vi "List Contents of Bucket.vi"() -> ()   [LabVIEW 2015]
doc: "This example shows you how to list the contents of your Amazon S3 bucket.\n\nThe list will contain information about all the objects you have in the bucket."
uses:
  <vilib>/AWS Toolkit/Core/HTTP Request/AWS Credentials.ctl
  <vilib>/AWS Toolkit/Core/HTTP Request/HTTP Request.lvclass
  <vilib>/AWS Toolkit/S3/Bucket/Bucket.lvclass
panel:
  in  "Bucket Name":string
  in  "Secret Key":string
  in  "Access Key":string
  out "Bucket Contents":i32(listbox)
  # "Overview: Demonstrates how to display the contents of an Amazon S3 bucket.\nRequirements: NI Cloud Toolkit for AWS and a registered Amazon AWS account\nInstructions:\n1. Specify the Access Key and Secret Key for your AWS account. You can create an account at http://aws.amazon.com.\n2. Specify a Bucket Name for the bucket you want to inspect.\n3. Run the VI. All of the contents of the specified bucket will be displayed in the Bucket Contents indicator."
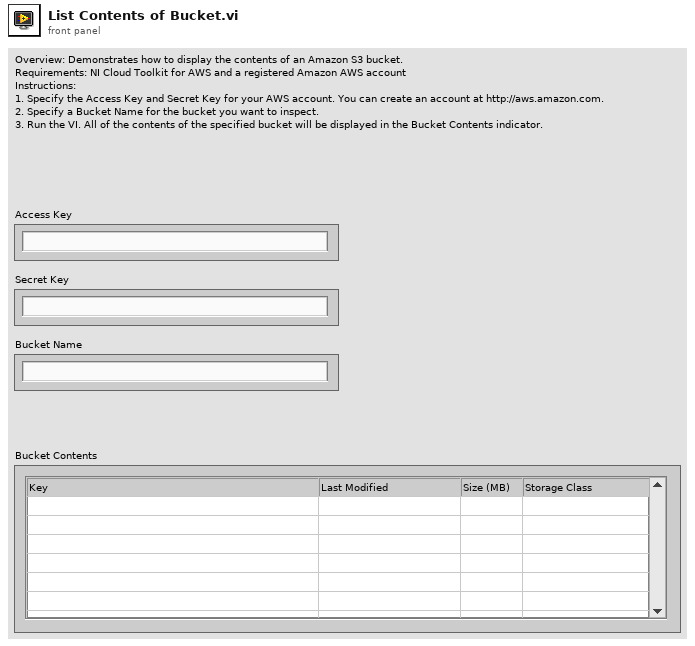
[diagram p1: front panel]
types:
  T1 = typedef "NI_AWS_Core.lvlib/HTTP Request.lvclass/AWS Credentials.ctl" = cluster{"Access Key":string, "Secret Key":string}
  T2 = typedef "NI_AWS_S3.lvlib/Object Content.ctl" = cluster{"Key":string, "Last Modified":timestamp, "ETag":string, "Size":u64, "Storage Class":T3, "Owner":T4}
  T3 = typedef "NI_AWS_S3.lvlib/Storage Class.ctl" = enum16{"STANDARD", "REDUCED_REDUNDANCY"}
  T4 = typedef "NI_AWS_S3.lvlib/Owner.ctl" = cluster{"ID":string, "Display Name":string}
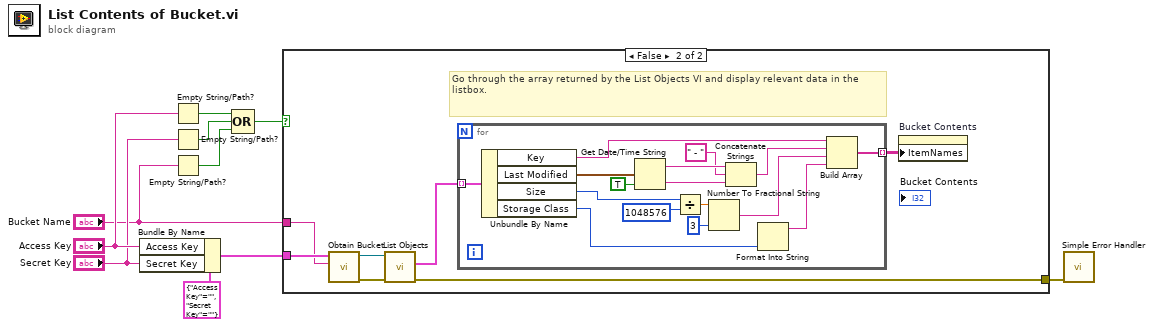
[diagram p0: block diagram]
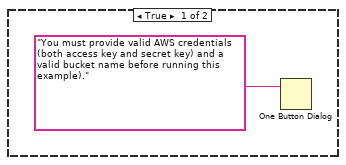
[diagram p2: hidden frame]
diagram:
  n1 = Bundle By Name(cluster=T1 {"Access Key"="", "Secret Key"=""} ("AWS Credentials in"), "Access Key"="Access Key", "Secret Key"="Secret Key") -> (w1:T1)
  n2 = Empty String/Path?(string/path="Access Key") -> (empty?=w9:bool)
  n3 = Empty String/Path?(string/path="Secret Key") -> (empty?=w8:bool)
  n4 = Empty String/Path?(string/path="Bucket Name") -> (empty?=w2:bool)
  n5 = Compound Arithmetic op=OR(w9, w8, w2) -> (w5:bool)
  n6 = case shown="False" w5 {
    tunnel: w1 -> [_ w15]
    tunnel: [_ w16] -> w4
    tunnel: "Bucket Name" -> [_ w13]
    frame True {
      n7 = One Button Dialog(message="You must provide valid AWS credentials (both access key and secret key) and a valid bucket name before running this example).") -> ()  [unwired: 1 in, 1 out]
    }
    frame False {
      # "Go through the array returned by the List Objects VI and display relevant data in the listbox."
      n8 = call <vilib>:"Obtain Bucket.vi"("Bucket name"=w13, "AWS Credentials"=w15) -> ("error out"=w14:errorcluster, "Bucket"=w12:refnum<class "Bucket.lvclass">)  [unwired: 8 in]
      n9 = call <vilib>:"List Objects.vi"("error in (no error)"=w14, "Bucket in"=w12) -> ("error out"=w16:errorcluster, "Objects"=w18:T2[])  [unwired: 6 in, 2 out]
      n10 = for {
        tunnel: w18 -> [w34] mode=indexing
        tunnel: [w19] -> w17 mode=indexing
        n11 = Unbundle By Name(w34) -> ("Key"=w23:string, "Last Modified"=w25:timestamp, "Size"=w33:u64, "Storage Class"=w24:T3)
        n12 = Get Date/Time String(seconds (now)=w25, want seconds? (F)=TRUE) -> (date string=w28:string, time string=w27:string)  [unwired: 1 in]
        n13 = Divide(x=w33, y=u64 1048576) -> (x/y=w31:dbl)
        n14 = Number To Fractional String(number=w31, precision (6)=i16 3) -> (F-format string=w21:string)  [unwired: 2 in]
        n15 = Concatenate Strings(w28, " - " ("string"), w27) -> (w22:string)
        n16 = Format Into String(w24) -> (resulting string=w20:string)  [unwired: 3 in, 1 out]
        n17 = Build Array(w23, w22, w21, w20) -> (w19:string[])
      }
      n18 = property on="Bucket Contents" class="MCListbox (strict)"("ItemNames"=w17) -> ()  [unwired: 2 in, 2 out]
    }
  }
  n19 = call <vilib>:"Simple Error Handler.vi"("error in (no error)"=w4) -> ()  [unwired: 4 in, 5 out]
